vi "deploy time report.vi"(6 "build_number":u32, 7 "test name":string, 8 "error in (no error)":errorcluster, 9 "timing":T1, 10 "workspace path":path, 11 "CLI in":refnum<class "CLI.lvclass">) -> (0 "error out":errorcluster, 3 "CLI out":refnum<class "CLI.lvclass">)   [LabVIEW 2014]
uses:
  <vilib>/Wiresmith Technology/LabVIEW CLI/CLI Class/CLI.lvclass
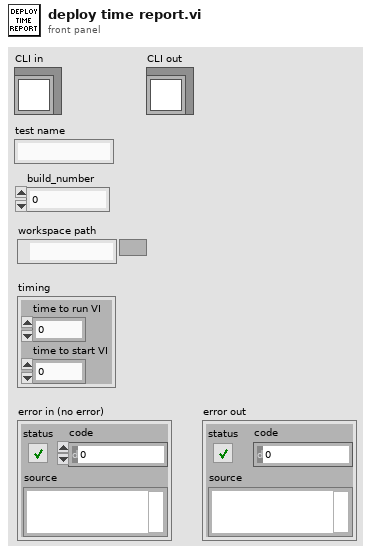
[diagram p1: front panel]
types:
  T1 = cluster{"time to run VI":u32, "time to start VI":u32}
  T2 = cluster{"time_to_deploy_run":u32, "time_to_start":u32, "test_name":string, "build_number":u32}
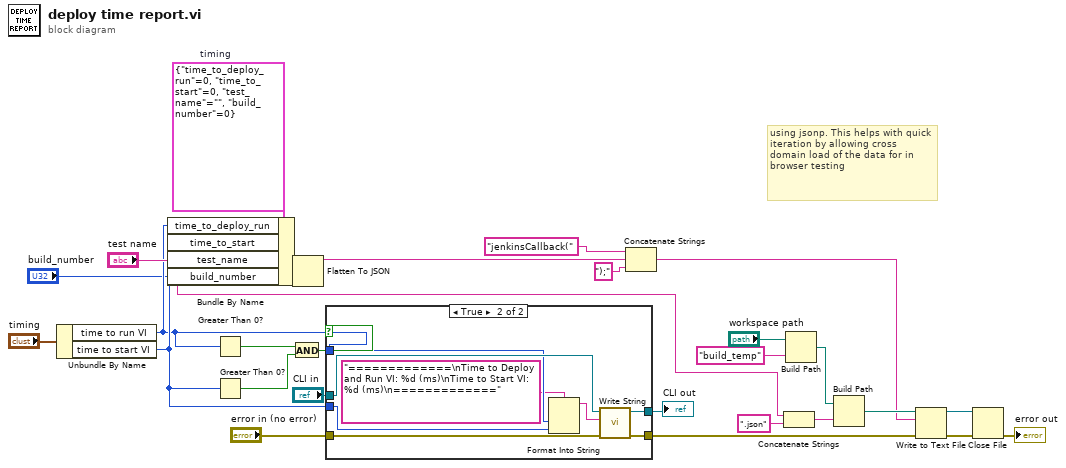
[diagram p0: block diagram]
diagram:
  w15 = T2 {"time_to_deploy_run"=0, "time_to_start"=0, "test_name"="", "build_number"=0}  # timing
  # "using jsonp. This helps with quick iteration by allowing cross domain load of the data for in browser testing"
  n1 = Unbundle By Name("timing") -> ("time to run VI"=w16:u32, "time to start VI"=w17:u32)
  n2 = Bundle By Name(cluster=w15, "time_to_deploy_run"=w16, "time_to_start"=w17, "test_name"="test name", "build_number"="build_number") -> (w18:T2)
  n3 = Greater Than 0?(x=w16) -> (x > 0?=w9:bool)
  n4 = Greater Than 0?(x=w17) -> (x > 0?=w8:bool)
  n5 = And(x=w9, y=w8) -> (x .and. y?=w10:bool)
  n6 = Flatten To JSON(anything=w18) -> (JSON string=w19:string)  [unwired: 2 in, 1 out]
  n7 = case shown="True" w10 {
    tunnel: "CLI in" -> [w29 w37]
    tunnel: [w29 w34] -> w12
    tunnel: "error in (no error)" -> [w28 w36]
    tunnel: [w28 w35] -> w3
    tunnel: w16 -> [_ w32]
    tunnel: w17 -> [_ w31]
    frame False {
    }
    frame True {
      n8 = Format Into String(format string="=============\nTime to Deploy and Run VI: %d (ms)\nTime to Start VI: %d (ms)\n=============", w32, w31) -> (resulting string=w33:string)  [unwired: 2 in, 1 out]
      n9 = call <vilib>:"Write String.vi"("error in (no error)"=w36, "Text to Write"=w33, "CLI in"=w37) -> ("error out"=w35:errorcluster, "CLI out"=w34:refnum<class "CLI.lvclass">)  [unwired: 7 in]
    }
  }
  "CLI out" <- w12
  n10 = Concatenate Strings("jenkinsCallback(" ("string"), w19, ");" ("string")) -> (w4:string)
  n11 = Concatenate Strings("test name", ".json" ("string")) -> (w24:string)
  n12 = Build Path(base path="workspace path", name or relative path="build_temp") -> (appended path=w27:path)
  n13 = Build Path(base path=w27, name or relative path=w24) -> (appended path=w5:path)
  n14 = Write to Text File(file (use dialog)=w5, text=w4, error in=w3) -> (refnum out=w7:refnum<file>, error out=w6:errorcluster)  [unwired: 1 in, 1 out]
  n15 = Close File(refnum=w7, error in=w6) -> (error out=→"error out":errorcluster)  [unwired: 1 out]
